vi "CheckRouteForSerialNumber.vi"(0 "class data in":refnum<class "CMESAPI.lvclass">, 5 "serialNumber":string, 7 "equipment":string, 9 "WorkorderNumber":string, 11 "error in (no error)":errorcluster) -> (4 "class data out":refnum<class "CMESAPI.lvclass">, 6 "Result":bool, 15 "error out":errorcluster)   [LabVIEW 2020, in "CMESAPI.lvlib" / "CMESAPI.lvclass"]
uses:
  CMESAPI.lvclass
  <vilib>/gpm_packages/@cs/event-logger/Source/Composed Log/Types/Log Level.ctl
  CMESAPI.lvclass/CMESAPI.ctl
  C:/Users/Fred Guo/Desktop/API_Salcomp_CMES/Libraries/CMESAPI/CMESAPI_Fw4.0_1.9.2/CMESAPI.dll
  CMESAPI_Fw4.0_1.9.2/CMESAPI.dll
  <vilib>/gpm_packages/@cs/event-logger/Source/Composed Log/LoggerReference/LoggerReference.lvclass/LoggerReference.ctl
  <vilib>/gpm_packages/@cs/event-logger/Source/Composed Log/LoggerReference/Log.vi
  <vilib>/gpm_packages/@cs/event-logger/Source/Composed Log/LoggerReference/Get Valid Event Time.vi
  <vilib>/gpm_packages/@cs/event-logger/Source/Composed Log/LoggerReference/Remove Stale Logs.vi
  <vilib>/gpm_packages/@cs/event-logger/Source/Composed Log/LoggerReference/LoggerReference.lvclass
  <vilib>/gpm_packages/@cs/event-logger/Source/Composed Log/Composed Log.lvlib
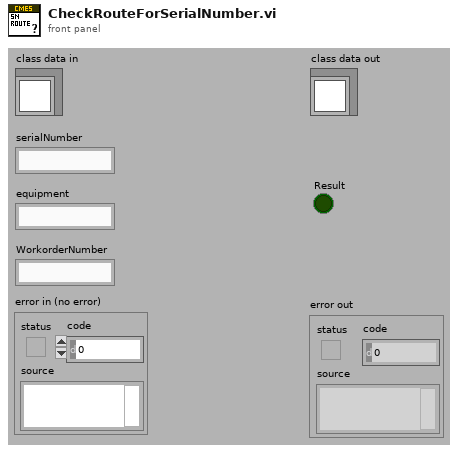
[diagram p1: front panel]
types:
  T1 = typedef "Composed Log.lvlib/Log Level.ctl" = enum16{"Debug", "Info", "Warning", "Error", "Critical"}
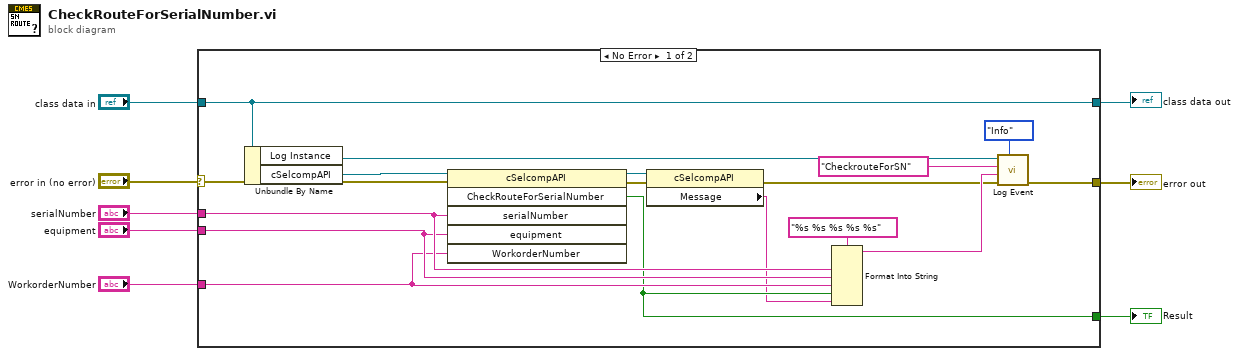
[diagram p0: block diagram]
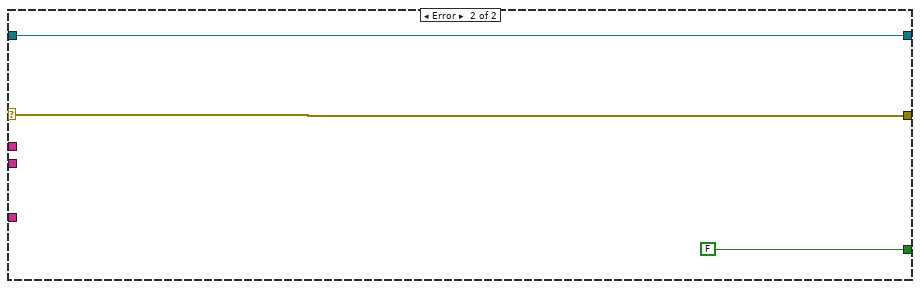
[diagram p2: hidden frame]
diagram:
  n1 = case shown="No Error" "error in (no error)" {
    selector: "error in (no error)" -> [w23 w28]
    tunnel: [w19 w28] -> w7
    tunnel: "class data in" -> [w25 w27]
    tunnel: [w25 w27] -> w5
    tunnel: "WorkorderNumber" -> [w15 _]
    tunnel: "equipment" -> [w16 _]
    tunnel: "serialNumber" -> [w17 _]
    tunnel: [w13 FALSE ("CheckRouteForSerialNumber")] -> w1
    frame No Error {
      n2 = Unbundle By Name(w25) -> ("Log Instance"=w18:refnum<class "LoggerReference.lvclass">, "cSelcompAPI"=w24:refnum<k24>)
      n3 = invoke on="Invoke Node" class="cSelcompAPI" method="CheckRouteForSerialNumber"(reference=w24, error in=w23, "serialNumber"=w17, "equipment"=w16, "WorkorderNumber"=w15) -> (reference out=w21:refnum<k24>, error out=w22:errorcluster, "CheckRouteForSerialNumber"=w13:bool)  [unwired: 1 in, 3 out]
      n4 = property class="cSelcompAPI"(reference=w21, error in=w22) -> (error out=w10:errorcluster, "Message"=w11:string)  [unwired: 1 out]
      n5 = Format Into String(format string="%s %s %s %s %s", w17, w16, w15, w13, w11) -> (resulting string=w12:string)  [unwired: 2 in, 1 out]
      n6 = call <vilib>:"Log Event.vi"("Event Level"=Log_Level."Info", "error in (no error)"=w10, "Data To Log"=w12, "SourceID"="CheckrouteForSN", "Log Instance"=w18) -> ("error out"=w19:errorcluster)  [unwired: 5 in, 1 out]
    }
    frame Error {
    }
  }
  "error out" <- w7
  "class data out" <- w5
  "Result" <- w1
